vi "LimitsV(SubVI).vi"(7 "Limits":dbl=1.1 format="%#_13g", 8 "RangeChB":T1(ring)=enum."10 В" caption="Диапазон \"B\"", 9 "RangeChA":T1(ring)=enum."10 В" caption="Диапазон \"A\"", 11 "Array":waveform(dbl)[](array[waveform])) -> (2 "x > y? 2":bool, 3 "x > y?":bool)   [LabVIEW 2017]
panel:
  out "Waveform Graph":waveform(dbl)[](graph)
  out "B":dbl
  out "A":dbl
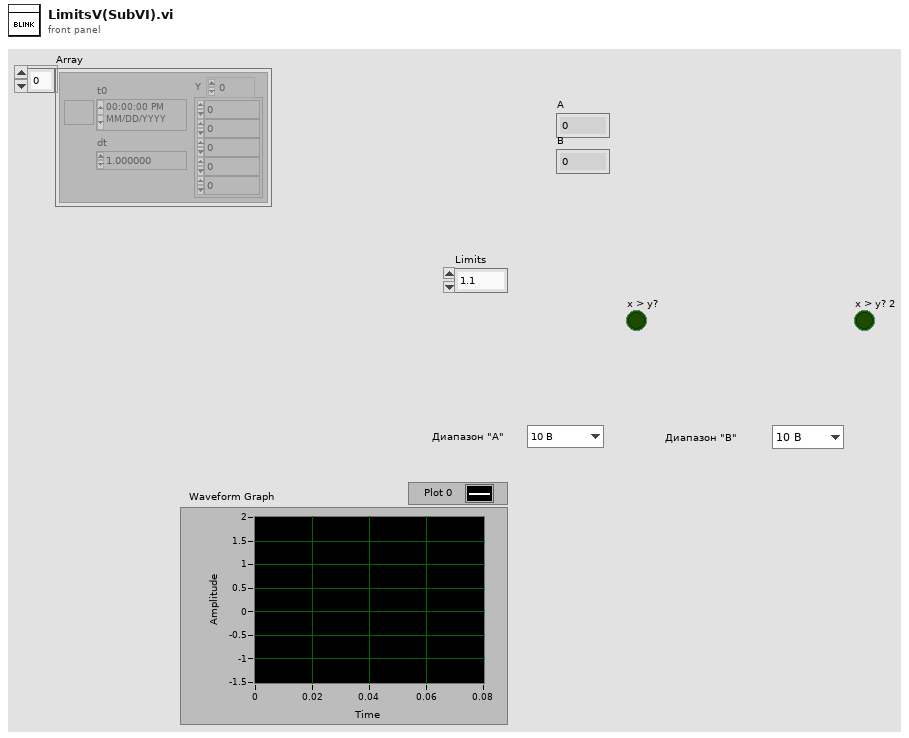
[diagram p1: front panel]
types:
  T1 = enum16{"5 мВ", "10 мВ", "25 мВ", "50 мВ", "100 мВ", "250 мВ", "0,5 В", "1,0 В", "2,5 В", "5 В", "10 В", "Авто", "Выкл."}
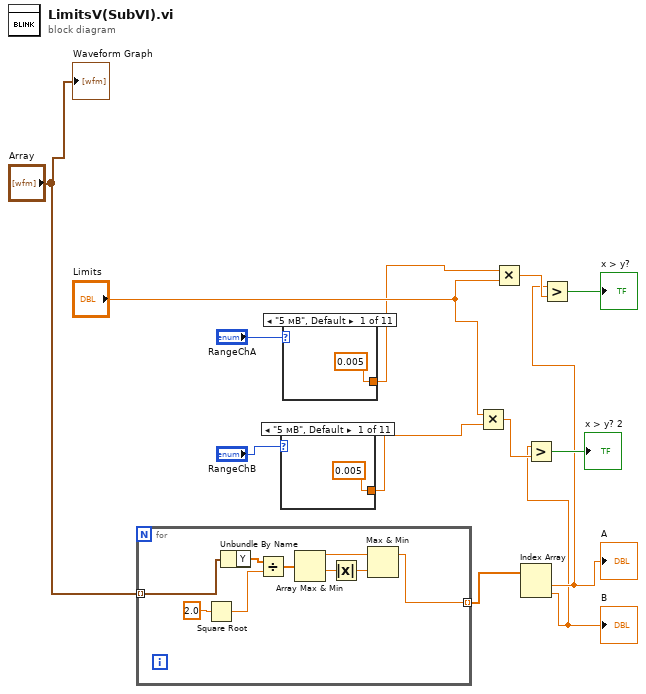
[diagram p0: block diagram]
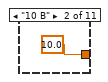
[diagram p2: hidden frame]
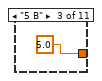
[diagram p3: hidden frame]
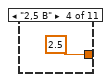
[diagram p4: hidden frame]
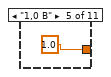
[diagram p5: hidden frame]
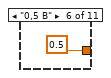
[diagram p6: hidden frame]
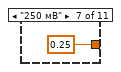
[diagram p7: hidden frame]
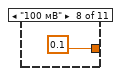
[diagram p8: hidden frame]
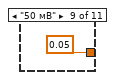
[diagram p9: hidden frame]
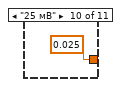
[diagram p10: hidden frame]
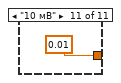
[diagram p11: hidden frame]
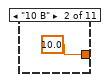
[diagram p12: hidden frame]
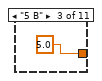
[diagram p13: hidden frame]
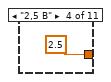
[diagram p14: hidden frame]
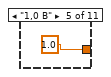
[diagram p15: hidden frame]
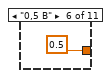
[diagram p16: hidden frame]
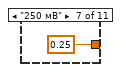
[diagram p17: hidden frame]
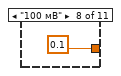
[diagram p18: hidden frame]
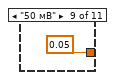
[diagram p19: hidden frame]
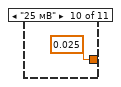
[diagram p20: hidden frame]
diagram:
  n1 = for {
    tunnel: "Array" -> [w15] mode=indexing
    tunnel: [w14] -> w3 mode=indexing
    n2 = Square Root(x=2.0) -> (sqrt(x)=w20:dbl)
    n3 = Unbundle By Name(w15) -> ("Y"=w22:dbl[])
    n4 = Divide(x=w22, y=w20) -> (x/y=w19:dbl[])
    n5 = Array Max & Min(array=w19) -> (max value=w16:dbl, min value=w17:dbl)  [unwired: 2 out]
    n6 = Absolute Value(x=w17) -> (abs(x)=w18:dbl)
    n7 = Max & Min(x=w16, y=w18) -> (max(x,y)=w14:dbl)  [unwired: 1 out]
  }
  n8 = case shown="\"5 мВ\", Default" "RangeChB" {
    tunnel: [0.005 10.0 5.0 2.5 1.0 0.5 0.25 0.1 0.05 0.025 0.01] -> w8
    frame "5 мВ", Default {
    }
    frame "10 В" {
    }
    frame "5 В" {
    }
    frame "2,5 В" {
    }
    frame "1,0 В" {
    }
    frame "0,5 В" {
    }
    frame "250 мВ" {
    }
    frame "100 мВ" {
    }
    frame "50 мВ" {
    }
    frame "25 мВ" {
    }
    frame "10 мВ" {
    }
  }
  n9 = case shown="\"5 мВ\", Default" "RangeChA" {
    tunnel: [0.005 10.0 5.0 2.5 1.0 0.5 0.25 0.1 0.05 0.025 0.01] -> w7
    frame "5 мВ", Default {
    }
    frame "10 В" {
    }
    frame "5 В" {
    }
    frame "2,5 В" {
    }
    frame "1,0 В" {
    }
    frame "0,5 В" {
    }
    frame "250 мВ" {
    }
    frame "100 мВ" {
    }
    frame "50 мВ" {
    }
    frame "25 мВ" {
    }
    frame "10 мВ" {
    }
  }
  n10 = Multiply(x="Limits", y=w8) -> (x*y=w5:dbl)
  n11 = Multiply(x=w7, y="Limits") -> (x*y=w6:dbl)
  n12 = Index Array(array=w3) -> (element #1=w2:dbl, element #2=w1:dbl)  [unwired: 2 in]
  "A" <- w2
  "B" <- w1
  n13 = Greater?(x=w1, y=w5) -> (0:→"x > y? 2":bool)
  n14 = Greater?(x=w2, y=w6) -> (0:→"x > y?":bool)
  "Waveform Graph" <- "Array"
